vi "Create Report.vi"(8 "error in (no error)":errorcluster, 11 "ZenReport configuration filepath":path) -> (0 "error out":errorcluster, 3 "ZenReport public data":T1)   [LabVIEW 2015]
uses:
  Typedefs/ZenReport private.ctl
  <vilib>/Utility/config.llb/Read Key (Boolean).vi
  <vilib>/Utility/config.llb/NI_LVConfig.lvlib
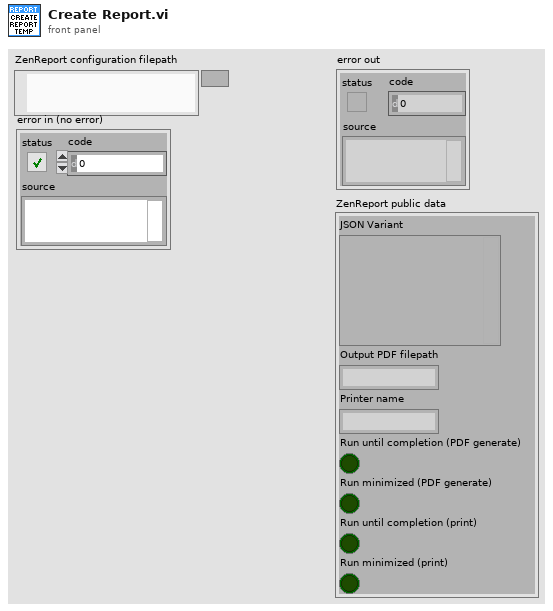
[diagram p1: front panel]
types:
  T1 = typedef "ZenReport private.ctl" = cluster{"JSON Variant":variant, "Output PDF filepath":string, "Printer name":string, "Run until completion (PDF generate)":bool, "Run minimized (PDF generate)":bool, "Run until completion (print)":bool, "Run minimized (print)":bool}
  T2 = typedef "NI_LVConfig.lvlib/Config Data RefNum.ctl" = refnum<k1>
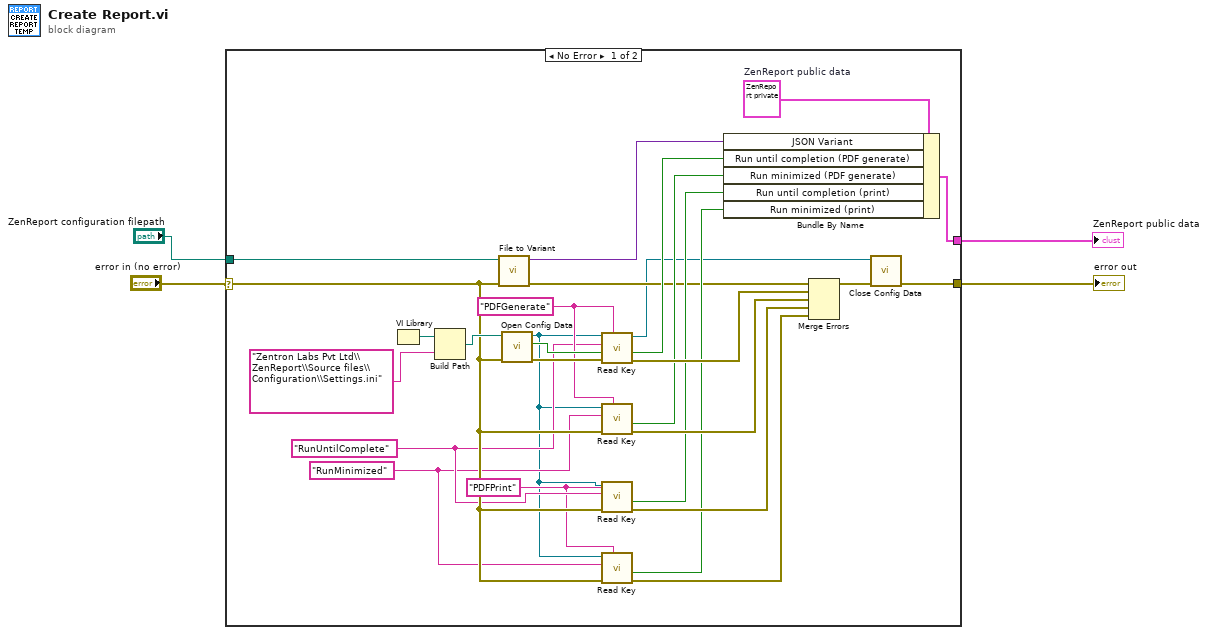
[diagram p0: block diagram]
diagram:
  n1 = case shown="No Error" "error in (no error)" {
    selector: "error in (no error)" -> [w16 w31]
    tunnel: [w28 _] -> w4
    tunnel: [w6 w31] -> w3
    tunnel: "ZenReport configuration filepath" -> [w17 _]
    frame No Error {
      w9 = "PDFPrint" ("section")
      w10 = "RunMinimized" ("key")
      w11 = "RunUntilComplete" ("key")
      w21 = "PDFGenerate" ("section")
      w30 = T1 {"JSON Variant"=variant, "Output PDF filepath"="", "Printer name"="", "Run until completion (PDF generate)"=FALSE, "Run minimized (PDF generate)"=FALSE, "Run until completion (print)"=FALSE, "Run minimized (print)"=FALSE}  # ZenReport public data
      n2 = VI Library() -> (path=w27:path)
      n3 = Build Path(base path=w27, name or relative path="Zentron Labs Pvt Ltd\\ZenReport\\Source files\\Configuration\\Settings.ini") -> (appended path=w25:path)
      n4 = call <vilib>:"File to Variant.vi"("JSON FilePath"=w17, "error in (no error)"=w16) -> ("JSON Variant"=w29:variant, "error out"=w7:errorcluster)  [unwired: 6 in, 1 out]
      n5 = call <vilib>:"Open Config Data.vi"("error in (no error)"=w16, "configuration file path"=w25) -> ("error out"=w24:errorcluster, "file created?"=w23:bool, "refnum"=w8:T2)  [unwired: 7 in]
      n6 = call-poly <vilib>:"Read Key.vi"("section"=w21, "error in (no error)"=w24, "default value"=w23, "key"=w11, "refnum"=w8) -> ("error out"=w22:errorcluster, "value"=w20:bool, "refnum out"=w5:T2)  [unwired: 3 in, 1 out]
      n7 = call-poly <vilib>:"Read Key.vi"("section"=w21, "error in (no error)"=w16, "key"=w10, "refnum"=w8) -> ("error out"=w18:errorcluster, "value"=w19:bool)  [unwired: 4 in, 2 out]
      n8 = call-poly <vilib>:"Read Key.vi"("section"=w9, "error in (no error)"=w16, "key"=w11, "refnum"=w8) -> ("error out"=w15:errorcluster, "value"=w13:bool)  [unwired: 4 in, 2 out]
      n9 = call-poly <vilib>:"Read Key.vi"("section"=w9, "error in (no error)"=w16, "key"=w10, "refnum"=w8) -> ("error out"=w14:errorcluster, "value"=w12:bool)  [unwired: 4 in, 2 out]
      n10 = Bundle By Name(cluster=w30, "JSON Variant"=w29, "Run until completion (PDF generate)"=w20, "Run minimized (PDF generate)"=w19, "Run until completion (print)"=w13, "Run minimized (print)"=w12) -> (w28:T1)
      n11 = Merge Errors(w7, w22, w18, w15, w14) -> ()  [unwired: 1 out]
      n12 = call <vilib>:"Close Config Data.vi"("error in (no error)"=w7, "refnum"=w5) -> ("error out"=w6:errorcluster)  [unwired: 8 in, 1 out]
    }
    frame Error {
    }
  }
  "error out" <- w3
  "ZenReport public data" <- w4
